vi "Moxom Run.vi"() -> ()   [LabVIEW 2011]
uses:
  <vilib>/Platform/TimedLoop/XDataNode/timing_clust.ctl
  <vilib>/Platform/TimedLoop/XDataNode/nitl_modes.ctl
  <vilib>/Platform/TimedLoop/XDataNode/wakeup.ctl
  <vilib>/Instr/_visa.llb/VISA Configure Serial Port (Instr).vi
  <vilib>/Utility/inputDevices.llb/joystickAcquire.vi
  <vilib>/Utility/inputDevices.llb/closeJoystick.vi
  <instrlib>/Hokuyo URG Series/Public/Initialize-Standard.vi
  <vilib>/Platform/TimedLoop/XDataNode/XDataNode.xnode
  <instrlib>/Hokuyo URG Series/Hokuyo URG Series.lvlib
  <vilib>/Platform/TimedLoop/XDataNode/XDNodeRunTimeDep.lvlib
panel:
  out "Motor control string":string="!M 0 16"
  out "Motor Remote":cluster{"Left Motor":dbl, "Right Motor":dbl}={"Left Motor"=0.0, "Right Motor"=16.0}
  out "Motor Auto":cluster{"Left Motor":dbl, "Right Motor":dbl}={"Left Motor"=200.0, "Right Motor"=500.0}
  out "Stop Robot":bool
  out "Turn Left":bool=TRUE
  out "Turn Right":bool
  in  "Lidar Serial Port":refnum<visa-resource-name>="COM20"
  out "Kill Switch Enabled":bool
  in  "Motor Controller\nSerial Port":refnum<visa-resource-name>="COM14"
  out "Auto Enabled":bool
  in  "Auto":bool
  in  "stop":bool
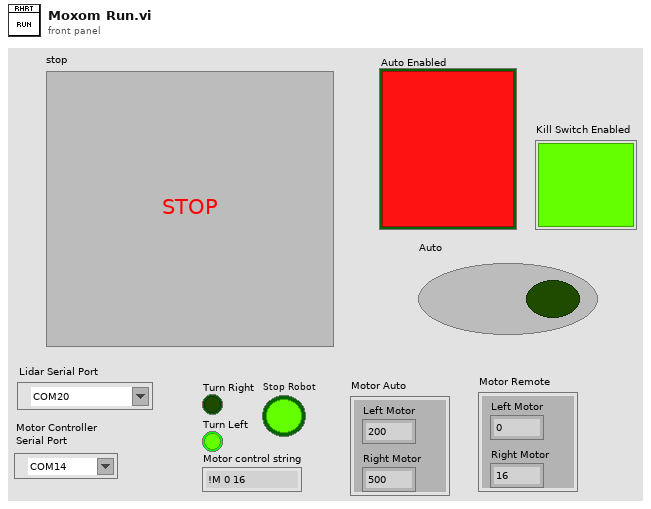
[diagram p1: front panel]
types:
  T1 = cluster{"axes total":u32, "buttons total":u32, "pov total":u32, "device name":string}[]
  T2 = cluster{"button 1":bool, "button 2":bool, "button 3":bool, "button 4":bool, "button 5":bool, "button 6":bool, "button 7":bool, "button 8":bool, "button 9":bool, "button 10":bool, "button 11":bool, "button 12":bool, "button 13":bool, "button 14":bool, "button 15":bool, "button 16":bool, "button 17":bool, "button 18":bool, "button 19":bool, "button 20":bool, "button 21":bool, "button 22":bool, "button 23":bool, "button 24":bool, "button 25":bool, "button 26":bool, "button 27":bool, "button 28":bool, "button 29":bool, "button 30":bool, "button 31":bool, "button 32":bool}
  T3 = typedef "XDNodeRunTimeDep.lvlib/timing_clust.ctl" = cluster{"Expected End [f-1]":u64, "Actual End [f-1]":u64, "Finished Late? [f-1]":bool, "Expected End [i-1]":u64, "Actual End [i-1]":u64, "Finished Late? [i-1]":bool, "Expected Start [i]":u64, "Actual Start [i]":u64, "Expected Start [f]":u64, "Actual Start [f]":u64, "Source Name":string, "Structure Name":string, "Period":i64, "Deadline":i64, "Offset":i64, "Start":i64, "Priority":i32, "Timeout":i32, "Mode":T4, "Wakeup Reason":T5, "Error":errorcluster, "Source Type":string, "Secondary Source Type":string, "Global End Time":u64, "Global Start Time":u64, "Frame Duration":u64, "Iteration Duration":u64, "Assigned CPU":i32, "I/O Scan Engine Mode":u32}
  T4 = typedef "XDNodeRunTimeDep.lvlib/nitl_modes.ctl" = enum32{"No Change", "Process missed periods, maintain original phase", "Discard missed periods, maintain original phase", "Process missed periods, ignore original phase", "Discard missed periods, ignore original phase"}
  T5 = typedef "XDNodeRunTimeDep.lvlib/wakeup.ctl" = enum32{"Normal", "Aborted", "Asynchronous wakeup", "Timing source error", "Timed loop error", "Timeout"}
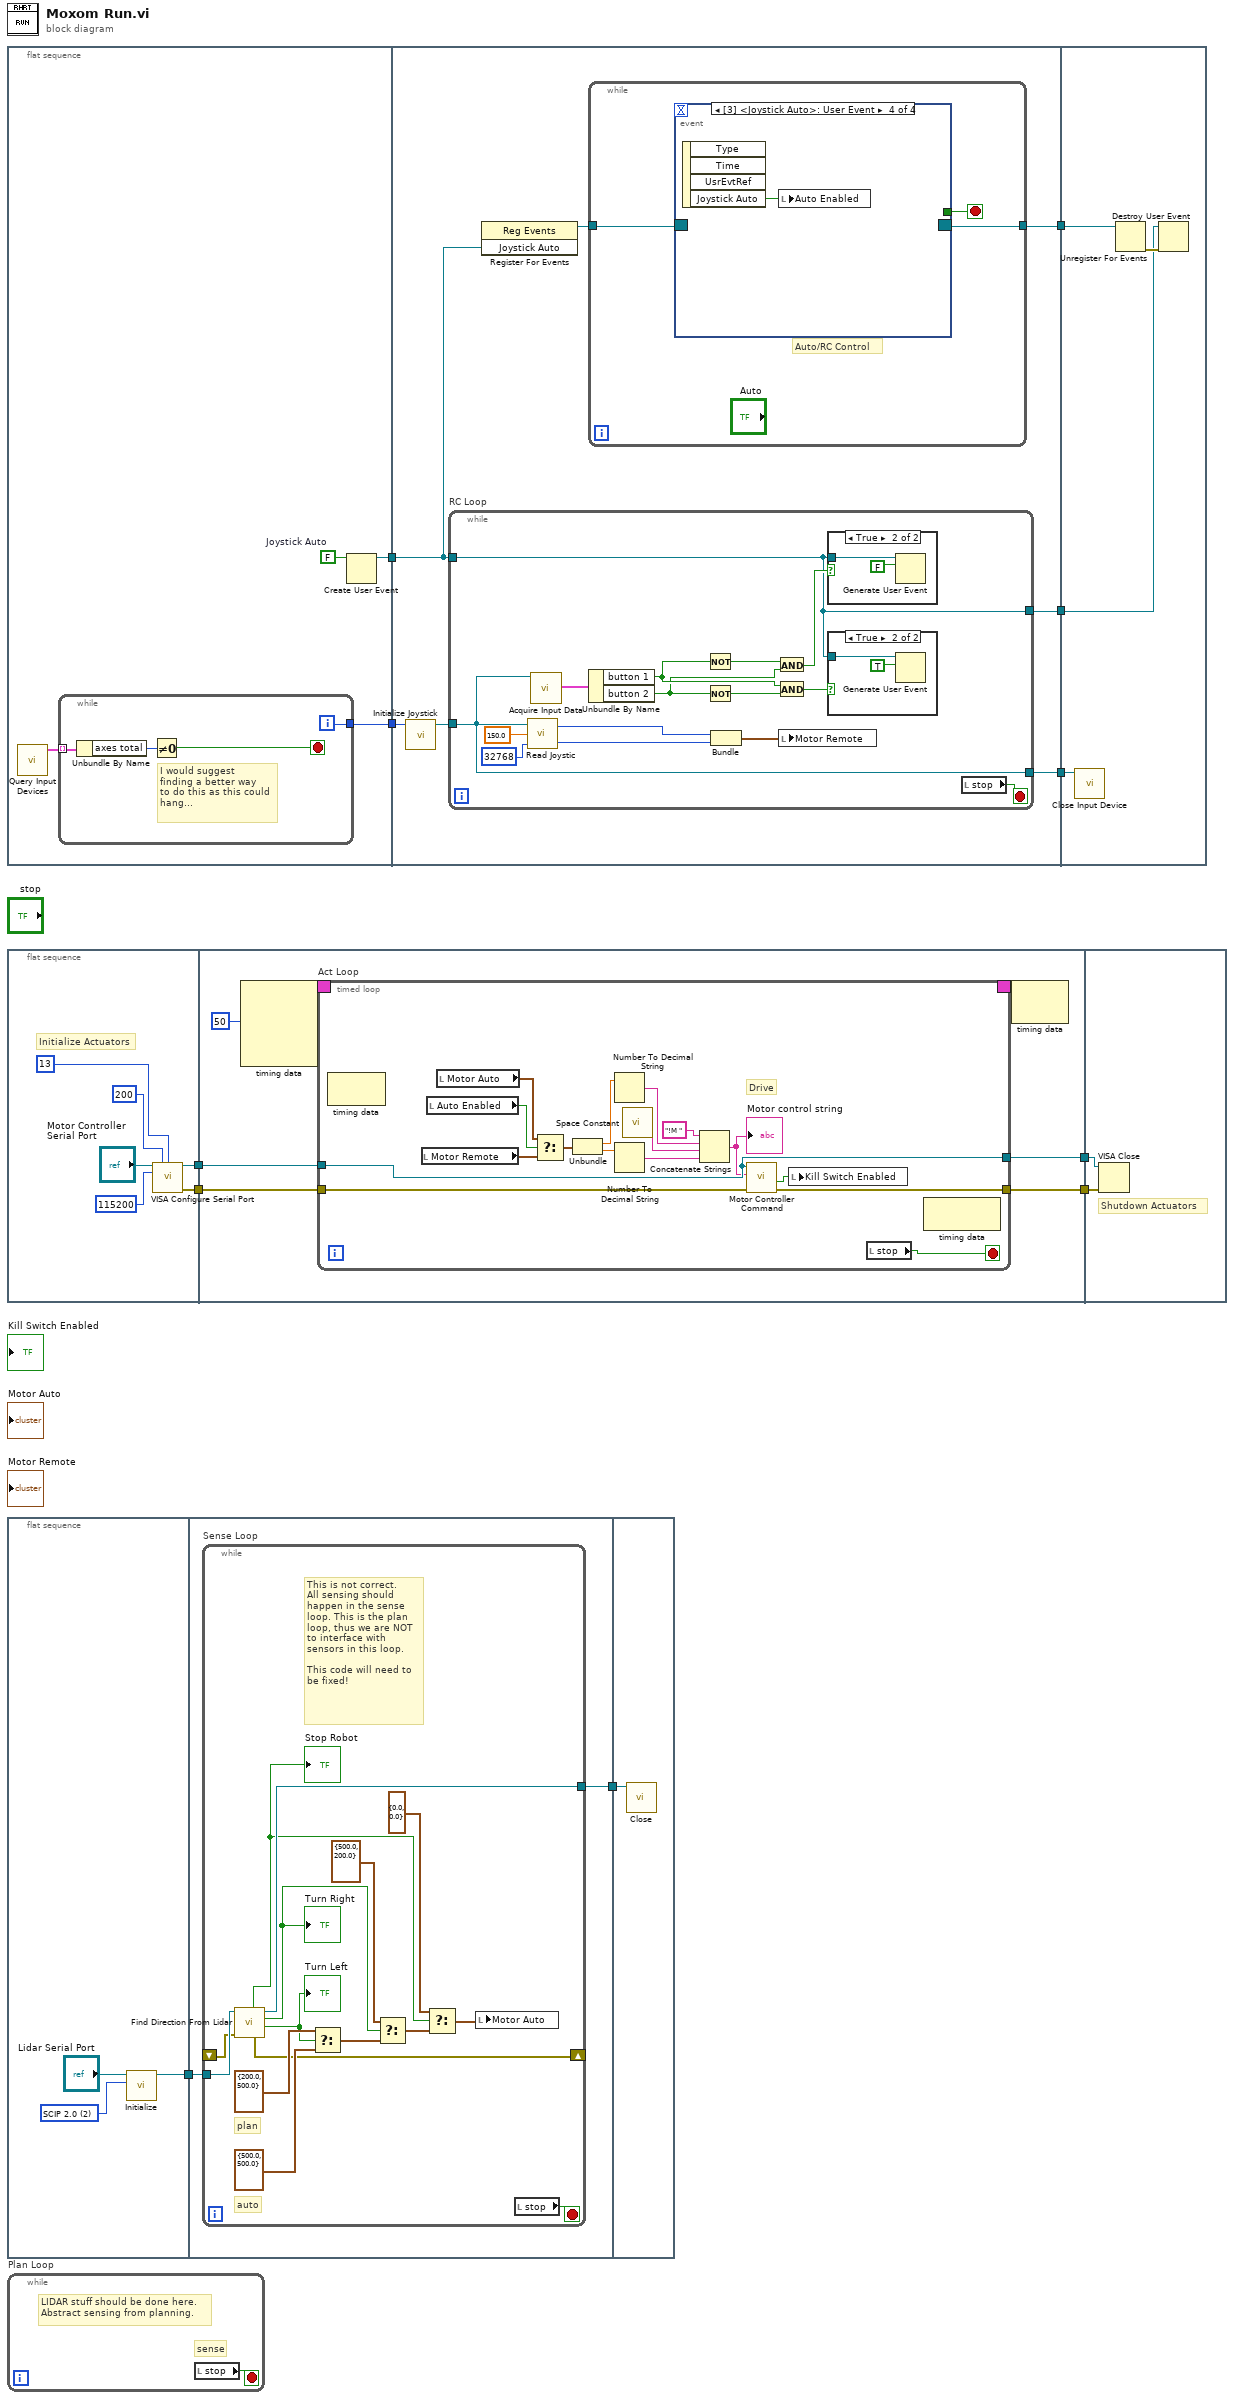
[diagram p0: block diagram]
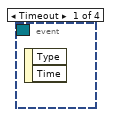
[diagram p4: hidden frame]
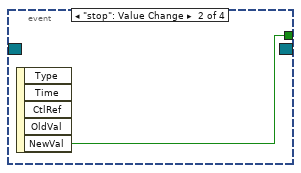
[diagram p5: hidden frame]
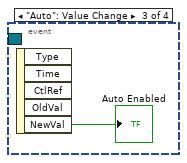
[diagram p6: hidden frame]
diagram:
  n1 = flat-sequence {
    tunnel: [w13] -> w10
    tunnel: [w12] -> w9
    tunnel: w10 -> [w24]
    tunnel: w9 -> [w23]
    tunnel: [w22] -> w8
    tunnel: [w21] -> w7
    tunnel: [w20] -> w6
    tunnel: w8 -> [w54]
    tunnel: w7 -> [w53]
    tunnel: w6 -> [w52]
    frame #0 {
      w14 = FALSE  # Joystick Auto
      n2 = call <vilib>:"Query Input Devices.vi"() -> ("joystick info"=w15:T1)  [unwired: 8 in, 3 out]
      n3 = while {
        tunnel: w15 -> [w19] mode=indexing
        tunnel: [w16] -> w12
        i -> [w16]
        stop <- w17 stop-if-true
        # "I would suggest\nfinding a better way\nto do this as this could\nhang..."
        n4 = Unbundle By Name(w19) -> ("axes total"=w18:u32)
        n5 = Not Equal To 0?(x=w18) -> (x != 0?=w17:bool)
      }
      n6 = Create User Event(user event datatype=w14) -> (user event=w13:refnum<user-event>)  [unwired: 1 in, 1 out]
    }
    frame #1 {
      n7 = call <vilib>:"Initialize Joystick.vi"("device index"=w23) -> ("device ID"=w25:refnum<k1>)  [unwired: 9 in, 1 out]
      n8 = while "RC Loop" {
        tunnel: w25 -> [w34]
        tunnel: [w34] -> w20
        tunnel: w24 -> [w27]
        tunnel: [w27] -> w22
        stop <- w41 stop-if-true
        n9 = call "Read Joystic.vi"("JoystickOutMaximum"=32768, "MaxMotorSpeed"=150.0 ("HalfMaxMotorSpeed"), "device ID"=w34) -> ("Right Motor"=w36:i32, "Left Motor"=w37:i32)
        n10 = call-poly <vilib>:"Acquire Input Data.vi"("device ID"=w34) -> ("button info"=w35:T2)  [unwired: 14 in, 4 out]
        n11 = Unbundle By Name(w35) -> ("button 1"=w31:bool, "button 2"=w30:bool)
        n12 = Not(x=w31) -> (.not. x?=w29:bool)
        n13 = Not(x=w30) -> (.not. x?=w28:bool)
        n14 = Bundle("Left Motor"=w37, "Right Motor"=w36) -> (w38:cluster{"Left Motor":i32, "Right Motor":i32})  [unwired: 1 in]
        n15 = And(x=w29, y=w30) -> (x .and. y?=w33:bool)
        n16 = And(x=w31, y=w28) -> (x .and. y?=w32:bool)
        n17 = local write "Motor Remote"(w38) -> ()
        n18 = case shown="True" w33 {
          tunnel: w27 -> [_ w42]
          frame False {
          }
          frame True {
            n19 = Generate User Event(user event=w42, event data cluster=FALSE ("Auto Enabled")) -> ()  [unwired: 1 in, 2 out]
          }
        }
        n20 = case shown="True" w32 {
          tunnel: w27 -> [_ w44]
          frame False {
          }
          frame True {
            n21 = Generate User Event(user event=w44, event data cluster=TRUE ("Auto Enabled")) -> ()  [unwired: 1 in, 2 out]
          }
        }
        n22 = local read "stop"() -> (w41:bool)
      }
      n23 = register-events(w24) -> (reference out=w26:refnum<event-registration>)  [unwired: 2 in, 1 out]
      n24 = while {
        tunnel: w26 -> [w47]
        tunnel: [w46] -> w21
        stop <- w48 stop-if-true
        # "Auto/RC Control"
        n25 = event shown="[3] <Joystick Auto>: User Event" {
          selector: w47 -> [_ _ _ _]
          dyn-events: [_ _ _ _] -> w46
          timeout: _ -> [_ _ _ _]
          tunnel: [_ w49 _ _] -> w48
          event Timeout {
            n26 = event-data() -> ()  [unwired: 1 in, 2 out]
          }
          event "stop": Value Change {
            n27 = event-data() -> ("NewVal"=w49:bool)  [unwired: 1 in, 4 out]
          }
          event "Auto": Value Change {
            n28 = event-data() -> ("NewVal"=→"Auto Enabled":bool)  [unwired: 1 in, 4 out]
          }
          event User Event {
            n29 = event-data() -> ("Joystick Auto"=w51:bool)  [unwired: 1 in, 3 out]
            n30 = local write "Auto Enabled"(w51) -> ()
          }
        }
      }
    }
    frame #2 {
      n31 = call-poly <vilib>:"Close Input Device.vi"("device ID"=w52) -> ()  [unwired: 9 in, 1 out]
      n32 = Unregister For Events(event registration refnum=w53) -> (error out=w55:errorcluster)  [unwired: 1 in]
      n33 = Destroy User Event(user event=w54, error in=w55) -> ()  [unwired: 1 out]
    }
  }
  n34 = flat-sequence {
    tunnel: [w57] -> w4
    tunnel: [w56] -> w3
    tunnel: [w67] -> w2
    tunnel: w4 -> [w68]
    tunnel: [w66] -> w1
    tunnel: w3 -> [w65]
    tunnel: w2 -> [w92]
    tunnel: w1 -> [w91]
    frame #0 {
      # "Initialize Actuators"
      n35 = call-poly "VISA Configure Serial Port"("VISA resource name"="Motor Controller\nSerial Port", "timeout (10sec)"=u32 200, "termination char\n(0xA = '\\n' = LF)"=u8 13 ("termination char\n(0xA = '\\n' = LF)"), "baud rate (9600)"=u32 115200) -> ("VISA resource name out"=w57:refnum<visa-resource-name>, "error out"=w56:errorcluster)  [unwired: 10 in]
    }
    frame #1 {
      n36 = node-c288(i64 50 ("Period")) -> (w64:T3)  [unwired: 3 in]
      n37 = timed-loop "Act Loop" {
        tunnel: w68 -> [w80]
        tunnel: [w80] -> w67
        tunnel: [w70] -> w66
        tunnel: w65 -> [w69]
        timing: w64 -> [_]
        timing-out: [_] -> w63
        stop <- w84 stop-if-true
        # "Drive"
        n38 = node-c288() -> ()  [unwired: 1 in, 1 out]
        n39 = local read "Motor Remote"() -> (w75:cluster{"Left Motor":dbl, "Right Motor":dbl})
        n40 = local read "Auto Enabled"() -> (w83:bool)
        n41 = local read "Motor Auto"() -> (w74:cluster{"Left Motor":dbl, "Right Motor":dbl})
        n42 = Select(t=w74, s=w83, f=w75) -> (s? t:f=w73:cluster{"Left Motor":dbl, "Right Motor":dbl})
        n43 = Unbundle(w73) -> ("Left Motor"=w72:dbl, "Right Motor"=w71:dbl)
        n44 = Number To Decimal String(number=w72) -> (decimal integer string=w78:string)  [unwired: 1 in]
        n45 = Number To Decimal String(number=w71) -> (decimal integer string=w77:string)  [unwired: 1 in]
        n46 = call <vilib>:"Space Constant.vi"() -> ("String"=w81:string)
        n47 = Concatenate Strings("!M " ("string"), w78, w81, w77) -> (w79:string)
        "Motor control string" <- w79
        n48 = call "Motor Controller Command.vi"("error in (no error)"=w69, "Command"=w79, "VISA resource name"=w80) -> ("error out"=w70:errorcluster, "Timeout on read"=w76:bool)  [unwired: 5 in, 2 out]
        n49 = local write "Kill Switch Enabled"(w76) -> ()
        n50 = local read "stop"() -> (w84:bool)
        n51 = node-c288() -> ()  [unwired: 1 in, 1 out]
      }
      n52 = node-c288(w63) -> ()  [unwired: 1 out]
    }
    frame #2 {
      # "Shutdown Actuators"
      n53 = VISA Close(VISA resource name=w92, error in (no error)=w91) -> ()  [unwired: 1 out]
    }
  }
  n54 = flat-sequence {
    tunnel: [w93] -> w5
    tunnel: [w97] -> w11
    tunnel: w5 -> [w96]
    tunnel: w11 -> [w113]
    frame #0 {
      w95 = u32 2 items=["Convert to Latest", "SCIP 1.1", "SCIP 2.0"] ("Protocol (2: SCIP 2.0)")
      n55 = call-poly <instrlib>:"Initialize.vi"("Protocol (2: SCIP 2.0)"=w95, "VISA resource name"="Lidar Serial Port") -> ("VISA resource name out"=w93:refnum<visa-resource-name>)  [unwired: 8 in, 1 out]
    }
    frame #1 {
      n56 = while "Sense Loop" {
        shift-right: [w104] -> _
        shift-left: _ -> [w98]
        tunnel: [w103] -> w97
        tunnel: w96 -> [w99]
        stop <- w112 stop-if-true
        # "This is not correct. \nAll sensing should\nhappen in the sense\nloop. This is the plan\nloop, thus we are NOT\nto interface with \nsensors in this loop.\n\nThis code will need to\nbe fixed!"
        # "auto"
        # "plan"
        n57 = call "Find Direction From Lidar.vi"("error in (no error)"=w98, "VISA resource name"=w99) -> ("Turn Left"=w100:bool, "Turn Right"=w101:bool, "VISA resource name out"=w103:refnum<visa-resource-name>, "error out"=w104:errorcluster, "Stop Robot"=w102:bool)  [unwired: 2 in, 3 out]
        "Turn Right" <- w101
        "Turn Left" <- w100
        "Stop Robot" <- w102
        n58 = Select(t=cluster{"Left Motor":dbl, "Right Motor":dbl} {"Left Motor"=200.0, "Right Motor"=500.0} ("Motor Remote"), s=w100, f=cluster{"Left Motor":dbl, "Right Motor":dbl} {"Left Motor"=500.0, "Right Motor"=500.0} ("Motor Remote")) -> (s? t:f=w108:cluster{"Left Motor":dbl, "Right Motor":dbl})
        n59 = Select(t=cluster{"Left Motor":dbl, "Right Motor":dbl} {"Left Motor"=500.0, "Right Motor"=200.0} ("Motor Remote"), s=w101, f=w108) -> (s? t:f=w109:cluster{"Left Motor":dbl, "Right Motor":dbl})
        n60 = Select(t=cluster{"Left Motor":dbl, "Right Motor":dbl} {"Left Motor"=0.0, "Right Motor"=0.0} ("Motor Remote"), s=w102, f=w109) -> (s? t:f=w111:cluster{"Left Motor":dbl, "Right Motor":dbl})
        n61 = local write "Motor Auto"(w111) -> ()
        n62 = local read "stop"() -> (w112:bool)
      }
    }
    frame #2 {
      n63 = call <instrlib>:"Close.vi"("VISA resource name"=w113) -> ()  [unwired: 10 in, 1 out]
    }
  }
  n64 = while "Plan Loop" {
    stop <- w114 stop-if-true
    # "LIDAR stuff should be done here.\nAbstract sensing from planning."
    # "sense"
    n65 = local read "stop"() -> (w114:bool)
  }
